vi "ExplorerTree Example.vi"() -> (0 "error out":errorcluster, 3 "Selection":path[](array[path]))   [LabVIEW 2019, in "SimpleDependencyInspector.lvlib" / "File Explorer.lvlib"]
doc: "This example gets the content of a folder and displays it in a tree control. Similar to file explorer windows, this sorts alphabetically by sub-directories then files. The file extension icons are returned as a custom symbols array to be referenced in the tree control. If a file icon is not found, this queries the operating system shell icon and keeps the glyph cached.\n\nCreated By: Ryan Pacini"
uses:
  File Explorer.lvlib
panel:
  in  "Folder Path":path
  in  "Tree":string[](tree)
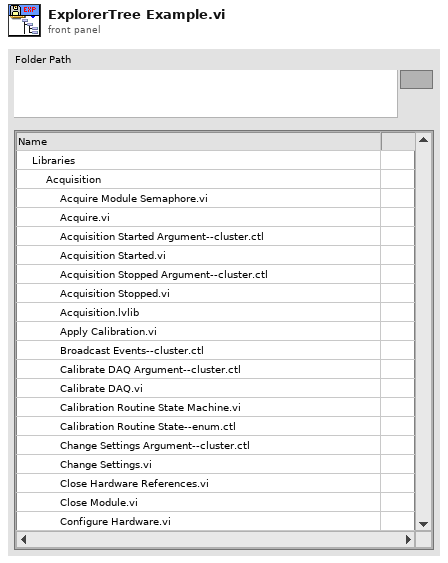
[diagram p1: front panel]
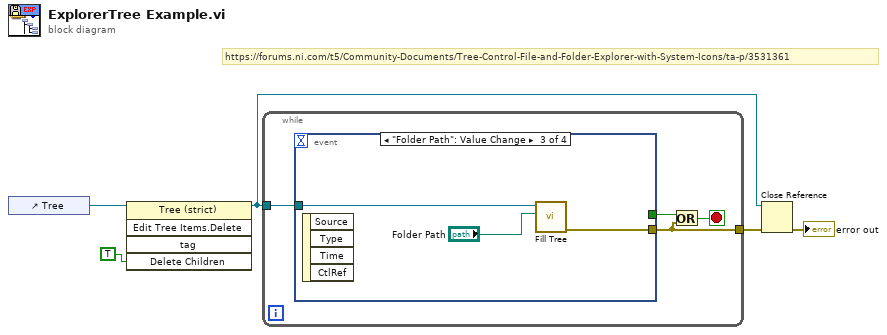
[diagram p0: block diagram]
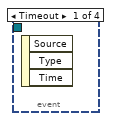
[diagram p2: hidden frame]
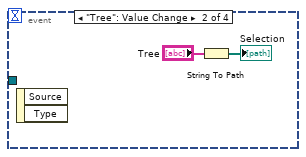
[diagram p3: hidden frame]
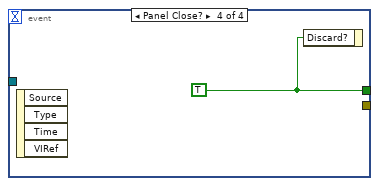
[diagram p4: hidden frame]
diagram:
  # "https://forums.ni.com/t5/Community-Documents/Tree-Control-File-and-Folder-Explorer-with-System-Icons/ta-p/3531361"
  n1 = control-ref of="Tree"() -> (w3:refnum<vi>)
  n2 = invoke class="Tree (strict)" method="Edit Tree Items.Delete"(reference=w3, "Delete Children"=TRUE ("Delete Children?")) -> (reference out=w2:refnum<vi>)  [unwired: 3 in, 4 out]
  n3 = while {
    tunnel: w2 -> [w7]
    tunnel: [w9] -> w5
    stop <- w6 stop-if-true
    n4 = event shown="[2] \"Folder Path\": Value Change" {
      selector: _ -> [_ _ _ _]
      dyn-events: _ -> [_ _ _ _]
      timeout: _ -> [_ _ _ _]
      tunnel: [_ _ _ w15] -> w8
      tunnel: w7 -> [_ _ w12 _]
      tunnel: [_ _ w14 _] -> w9
      event Timeout {
        n5 = event-data() -> ()  [unwired: 1 in, 3 out]
      }
      event "Tree": Value Change {
        n6 = event-data() -> ()  [unwired: 1 in, 2 out]
        n7 = String To Path(string="Tree") -> (path=→"Selection":path[])
      }
      event "Folder Path": Value Change {
        n8 = event-data() -> ()  [unwired: 1 in, 4 out]
        n9 = call "Fill Tree.vi"("Folder Path"="Folder Path", "TreeControl in"=w12) -> ("error out"=w14:errorcluster)  [unwired: 9 in]
      }
      event Panel Close? {
        w15 = TRUE ("Discard?")
        n10 = event-data() -> ()  [unwired: 1 in, 4 out]
        n11 = event-data("Discard?"=w15) -> ()  [unwired: 1 in, 1 out]
      }
    }
    n12 = Or(x=w8, y=w9) -> (x .or. y?=w6:bool)
  }
  n13 = Close Reference(reference=w2, error in (no error)=w5) -> (error out=→"error out":errorcluster)
